vi "W1Q2.vi"() -> ()   [LabVIEW 2021]
panel:
  out "seconds":dbl
  out "mins":dbl
  out "hrs":dbl
  in  "Numeric":dbl
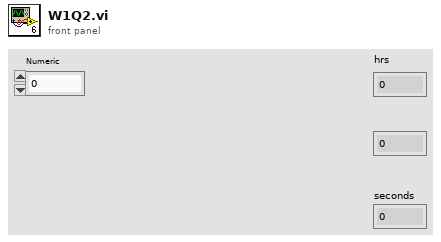
[diagram p1: front panel]
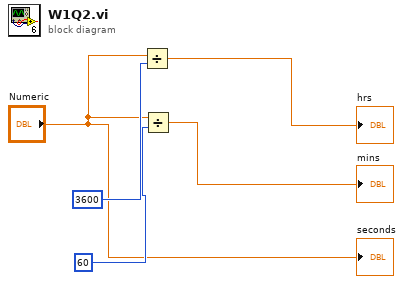
[diagram p0: block diagram]
diagram:
  n1 = Divide(x="Numeric", y=3600) -> (x/y=→"hrs":dbl)
  n2 = Divide(x="Numeric", y=60) -> (x/y=→"mins":dbl)
  "seconds" <- "Numeric"
